vi "Single HWSync.vi"() -> ()   [LabVIEW 2014]
doc: "Use this template to build a producer/consumer design pattern with events to produce queue items. Use this design pattern instead of the User Interface Event Handler pattern for user interfaces when you want to execute code asynchronously in response to an event without slowing the user interface responsiveness."
uses:
  TypeDefs/HAL Config Data.ctl
  APIs/Data Queue/Acquisition Data 1 Sample Cluster.ctl
  APIs/Data Queue/Control Data Cluster.ctl
  APIs/Message Queue/Enqueue Message (Array).vi
  APIs/Message Queue/WINFAS 2 Message Queue.lvlib
  HWSyncLoop/HWSyncLoop.lvlib
  APIs/Data Queue/WINFAS 2 Data Queue.lvlib
panel:
  in  "Config":bool
  in  "LOAD DRIVER":bool
  in  "Disconnect":bool
  in  "Connect":bool
  in  "Sequence:Stop":bool
  in  "Sequence:Start":bool
  in  "Auto-Refresh:Stop":bool
  in  "Auto-Refresh:Start":bool
  in  "Stop Cycle":bool
  in  "Stop Measurement":bool
  in  "Start Measurement":bool
  in  "Start Cycle":bool
  out "TDX":sgl[][](graph)
  out "Valores TDX":sgl[](array[numeric]) format="%0+10.6fmm"
  out "TDX N°":i32[](array[numeric])
  in  "Encoder Zero":bool
  out "DO":bool[][](array[boolean])
  out "DI":bool[][](array[boolean])
  in  "DO Button":bool[][](array[boolean])=[[FALSE, FALSE, FALSE, FALSE, FALSE, FALSE, FALSE, FALSE], [FALSE, FALSE, FALSE, FALSE, FALSE, FALSE, FALSE, FALSE]]
  out "Encoder":sgl(knob) scale=-360.0..360.0 scale format="%.0f°"
  out "Errores":string
  out "Status Bar":string="LOAD"
  out "Driver:":string
  # "Loop para 1 Hardware Síncrono"
  # "Entradas Digitales (0-15)"
  # "Salidas Digitales (0-15)"
  # "Salidas Digitales (0-15)"
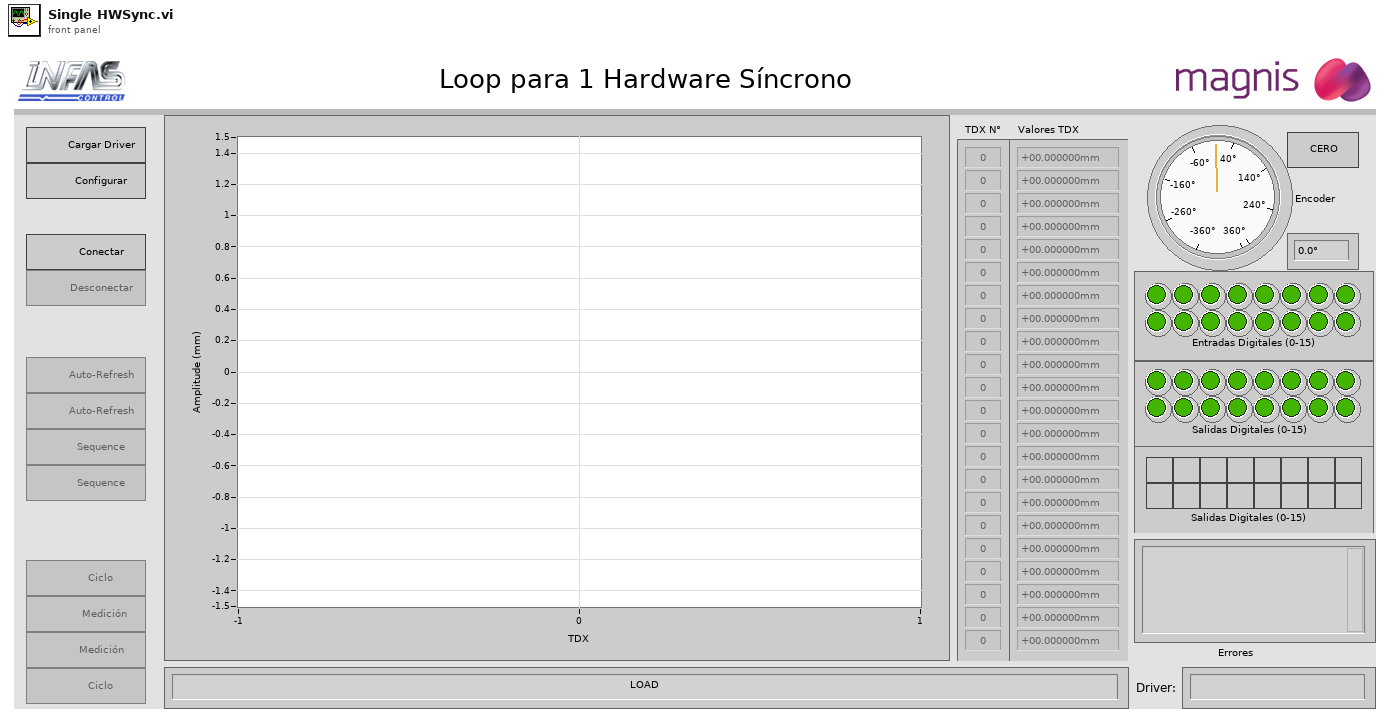
[diagram p1: front panel]
types:
  T1 = typedef "HAL Config Data.ctl" = cluster{"HWSync Index":u32, "Driver Name":string, "Channel Mask":u64}
  T2 = enum8{"Enabled", "Disabled", "Disabled and Grayed Out"}
  T3 = cluster{"LOAD DRIVER":refnum<vi>, "Config":refnum<vi>, "Connect":refnum<vi>, "Disconnect":refnum<vi>, "Auto-Refresh:Start":refnum<vi>, "Auto-Refresh:Stop":refnum<vi>, "Sequence:Start":refnum<vi>, "Sequence:Stop":refnum<vi>, "Start Cycle":refnum<vi>, "Start Measurement":refnum<vi>, "Stop Measurement":refnum<vi>, "Stop Cycle":refnum<vi>}
  T4 = enum32{"invalid app kind", "Development System", "Run Time System", "Student Edition", "Embedded LabVIEW", "Evaluation", "Custom"}
  T5 = typedef "WINFAS 2 Message Queue.lvlib/All Message Queues.ctl" = cluster{"CORE":refnum<queue>, "Event UI":refnum<queue>, "Display UI":refnum<queue>, "MATH":refnum<queue>, "SEQ":refnum<queue>, "DB":refnum<queue>, "ERR":refnum<queue>, "HAL":refnum<queue>, "HWSync1":refnum<queue>, "HWSync2":refnum<queue>, "HWSync3":refnum<queue>, "HWSync4":refnum<queue>, "HWSync5":refnum<queue>, "HWAsync1":refnum<queue>, "HWAsync2":refnum<queue>, "HWAsync3":refnum<queue>, "HWAsync4":refnum<queue>, "HWAsync5":refnum<queue>, "HWAsync6":refnum<queue>, "HWAsync7":refnum<queue>, "HWAsync8":refnum<queue>, "HWAsync9":refnum<queue>, "HWAsync10":refnum<queue>}
  T6 = typedef "WINFAS 2 Data Queue.lvlib/All Data Queues Cluster.ctl" = cluster{"Queues":cluster{"ACQ HWSync1":refnum<queue>, "ACQ HWSync2":refnum<queue>, "ACQ HWSync3":refnum<queue>, "ACQ HWSync4":refnum<queue>, "ACQ HWSync5":refnum<queue>}, "Notifiers":cluster{"Control":cluster{"CTRL HWSync1":refnum<notifier>, "CTRL HWSync2":refnum<notifier>, "CTRL HWSync3":refnum<notifier>, "CTRL HWSync4":refnum<notifier>, "CTRL HWSync5":refnum<notifier>}, "Acquisition":cluster{"ACQ HWSync1":refnum<notifier>, "ACQ HWSync2":refnum<notifier>, "ACQ HWSync3":refnum<notifier>, "ACQ HWSync4":refnum<notifier>, "ACQ HWSync5":refnum<notifier>}, "Async":cluster{"ACQ HWAsync1":refnum<notifier>, "ACQ HWAsync2":refnum<notifier>, "ACQ HWAsync3":refnum<notifier>, "ACQ HWAsync4":refnum<notifier>, "ACQ HWAsync5":refnum<notifier>, "ACQ HWAsync6":refnum<notifier>, "ACQ HWAsync7":refnum<notifier>, "ACQ HWAsync8":refnum<notifier>, "ACQ HWAsync9":refnum<notifier>, "ACQ HWAsync10":refnum<notifier>}}}
  T7 = typedef "WINFAS 2 Data Queue.lvlib/Acquisition Data 1 Sample Cluster.ctl" = cluster{"TDX":sgl[], "Encoder":sgl}
  T8 = typedef "WINFAS 2 Data Queue.lvlib/Control Data Cluster.ctl" = cluster{"Encoder":sgl, "DI":bool[], "DO":bool[]}
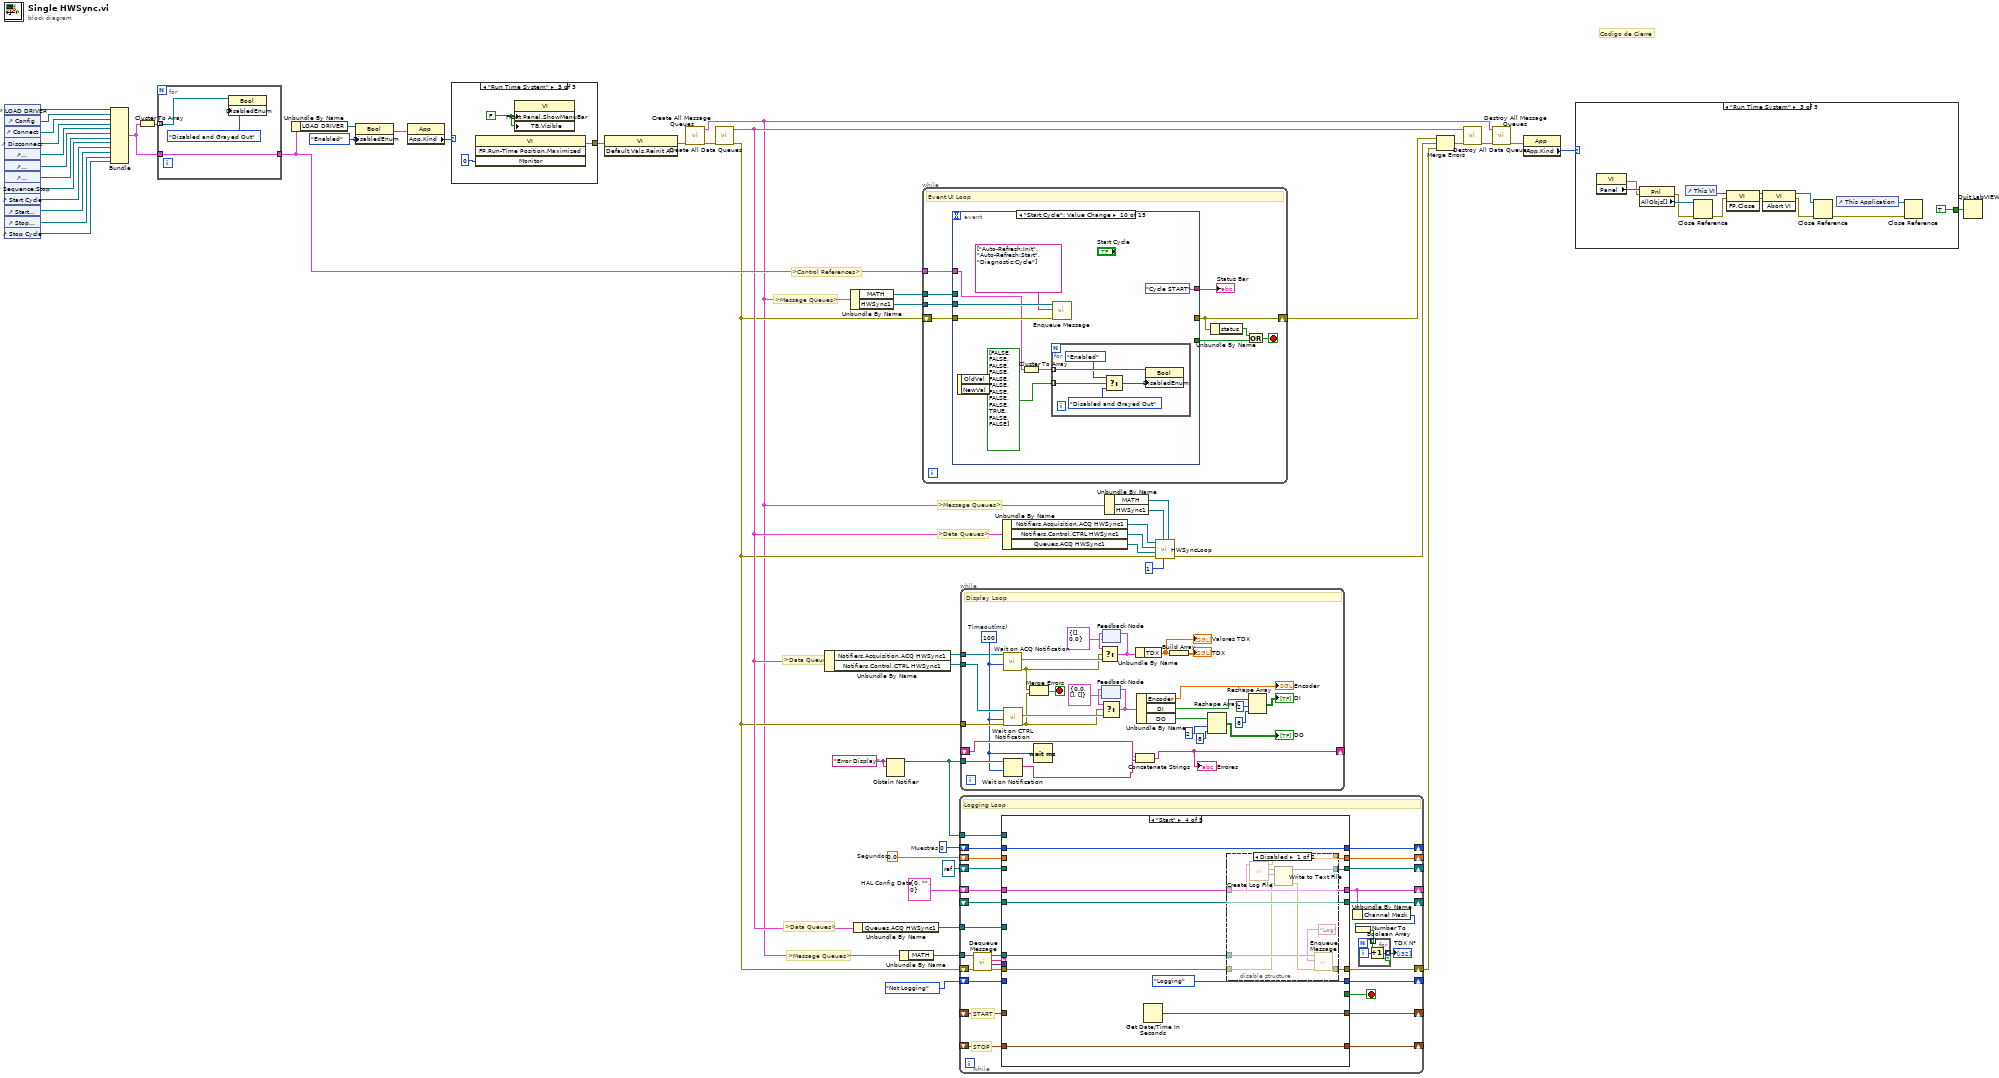
[diagram p0: block diagram]
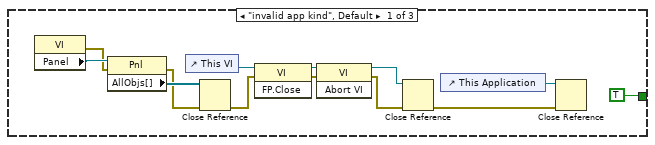
[diagram p4: hidden frame]
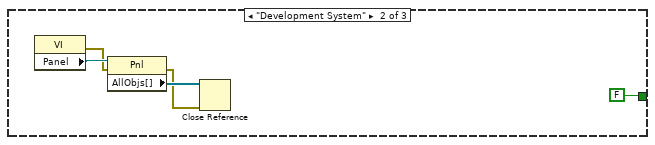
[diagram p5: hidden frame]
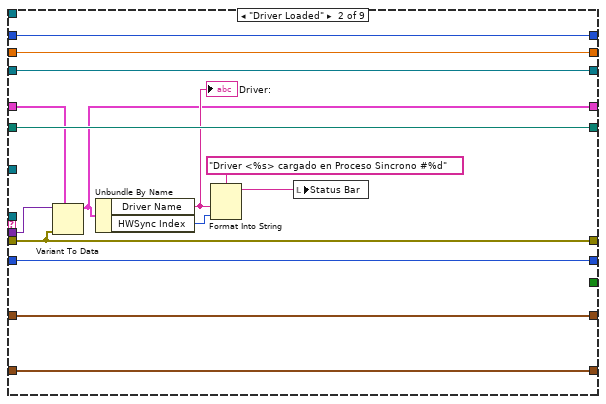
[diagram p7: hidden frame]
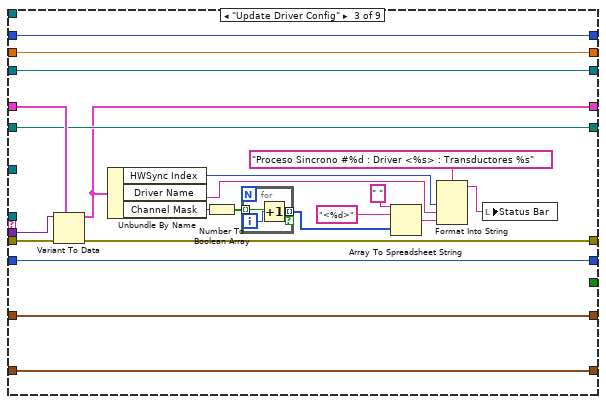
[diagram p8: hidden frame]
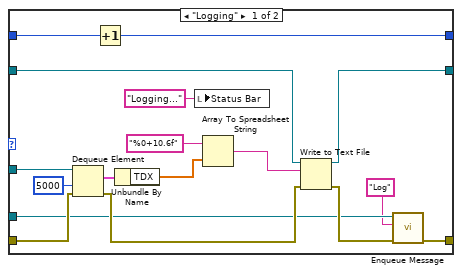
[diagram p11: hidden frame]
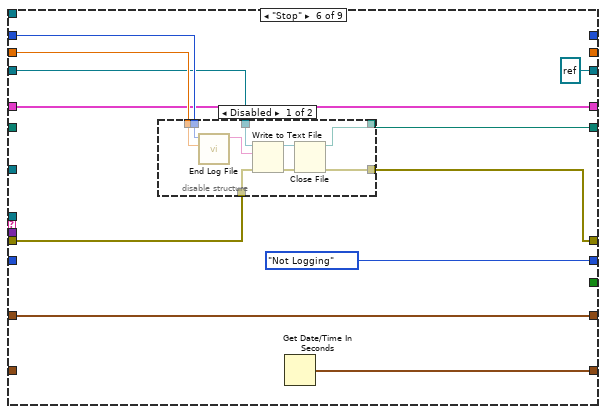
[diagram p12: hidden frame]
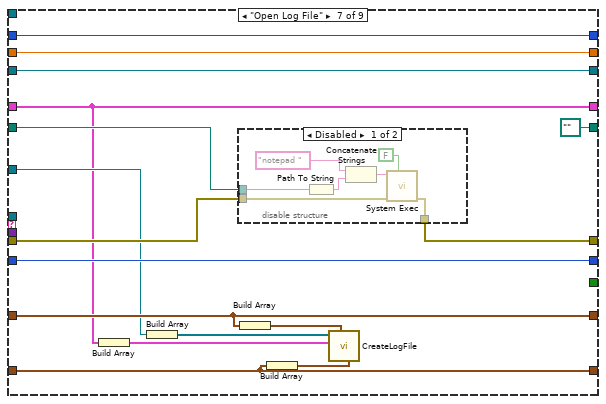
[diagram p14: hidden frame]
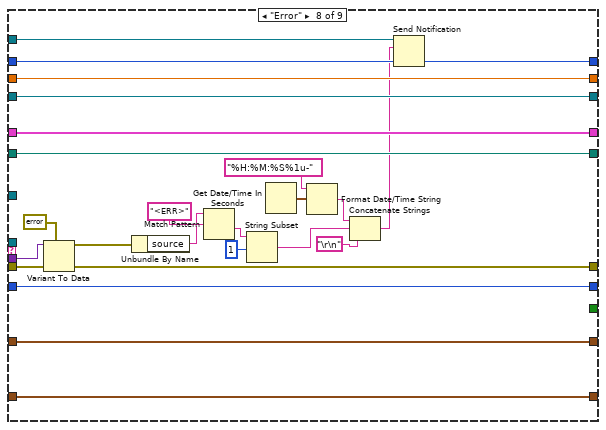
[diagram p16: hidden frame]
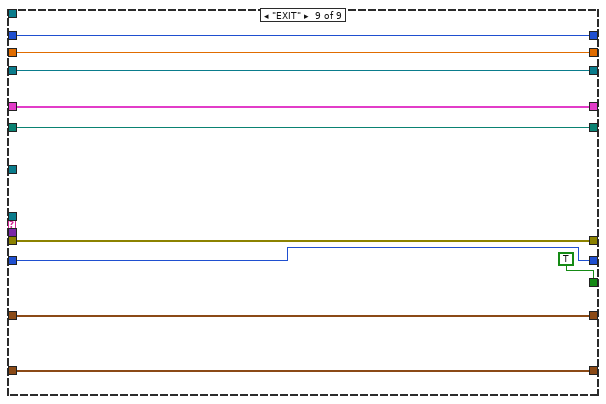
[diagram p17: hidden frame]
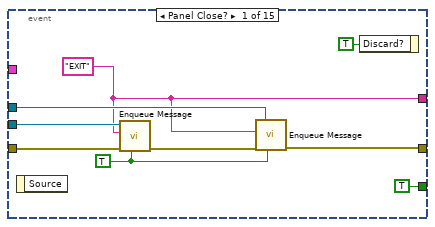
[diagram p18: hidden frame]
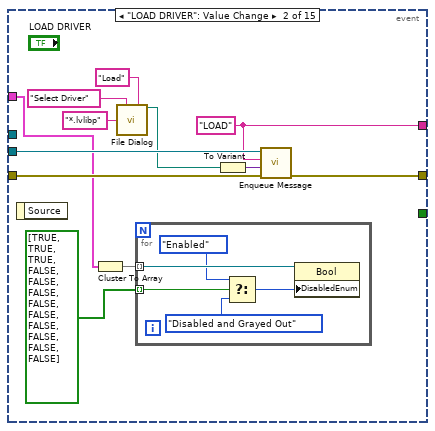
[diagram p19: hidden frame]
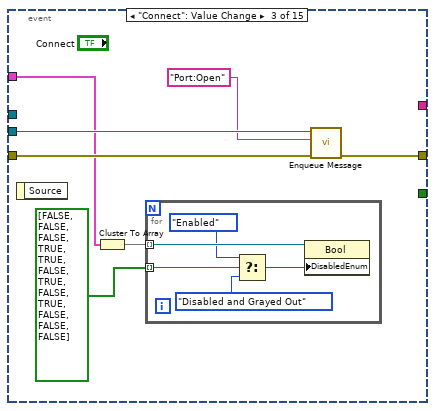
[diagram p20: hidden frame]
diagram:
  w2 = "Error Display" ("name (unnamed)")
  w11 = T1 {"HWSync Index"=0, "Driver Name"="", "Channel Mask"=0}  # HAL Config Data
  w43 = 0.0  # Segundos
  w44 = 0  # Muestras
  # ">Control References>"
  # "Codigo de Cierre"
  # ">Message Queues>"
  # ">Data Queues>"
  # ">Message Queues>"
  # ">Data Queues>"
  # ">Data Queues>"
  # ">Message Queues>"
  n1 = control-ref of="LOAD DRIVER"() -> (w14:refnum<vi>)
  n2 = control-ref of="Config"() -> (w8:refnum<vi>)
  n3 = control-ref of="Connect"() -> (w9:refnum<vi>)
  n4 = control-ref of="Disconnect"() -> (w10:refnum<vi>)
  n5 = control-ref of="Auto-Refresh:Start"() -> (w41:refnum<vi>)
  n6 = control-ref of="Auto-Refresh:Stop"() -> (w40:refnum<vi>)
  n7 = control-ref of="Sequence:Start"() -> (w39:refnum<vi>)
  n8 = control-ref of="Sequence:Stop"() -> (w38:refnum<vi>)
  n9 = control-ref of="Start Cycle"() -> (w6:refnum<vi>)
  n10 = control-ref of="Start Measurement"() -> (w5:refnum<vi>)
  n11 = control-ref of="Stop Measurement"() -> (w4:refnum<vi>)
  n12 = control-ref of="Stop Cycle"() -> (w3:refnum<vi>)
  n13 = Bundle("LOAD DRIVER"=w14, "Config"=w8, "Connect"=w9, "Disconnect"=w10, "Auto-Refresh:Start"=w41, "Auto-Refresh:Stop"=w40, "Sequence:Start"=w39, "Sequence:Stop"=w38, "Start Cycle"=w6, "Start Measurement"=w5, "Stop Measurement"=w4, "Stop Cycle"=w3) -> (w36:T3)  [unwired: 1 in]
  n14 = Cluster To Array(cluster=w36) -> (array=w37:refnum<vi>[])
  n15 = for {
    tunnel: w37 -> [w55] mode=indexing
    tunnel: w36 -> [w54]
    tunnel: [w54] -> w35
    n16 = property class="Bool"(reference=w55, "DisabledEnum"=T2."Disabled and Grayed Out" ("Disabled")) -> ()  [unwired: 1 in, 2 out]
  }
  n17 = Unbundle By Name(w35) -> ("LOAD DRIVER"=w34:refnum<vi>)
  n18 = property class="Bool"(reference=w34, "DisabledEnum"=T2."Enabled" ("Disabled")) -> (error out=w22:errorcluster)  [unwired: 1 in, 1 out]
  n19 = property class="App"(error in=w22) -> ("App.Kind"=w30:T4)  [unwired: 1 in, 2 out]
  n20 = case shown="\"Run Time System\"" w30 {
    tunnel: [_ _ w57] -> w29
    frame "invalid app kind", Default {
    }
    frame "Development System" {
    }
    frame "Run Time System" {
      w56 = FALSE ("Front Panel Window:Show Menu Bar")
      n21 = invoke class="VI" method="FP.Run-Time Position.Maximized"("Monitor"=i16 0) -> (error out=w57:errorcluster)  [unwired: 3 in, 3 out]
      n22 = property class="VI"("Front Panel.ShowMenuBar"=w56, "TB.Visible"=w56) -> ()  [unwired: 2 in, 2 out]
    }
  }
  n23 = invoke class="VI" method="Default Vals.Reinit All"(error in=w29) -> (error out=w16:errorcluster)  [unwired: 2 in, 2 out]
  n24 = call "Create All Message Queues.vi"("error in (no error)"=w16) -> ("error out"=w18:errorcluster, "Message Queues Out"=w12:T5)  [unwired: 9 in]
  n25 = call "Create All Data Queues.vi"("Error In"=w18) -> ("Error Out"=w13:errorcluster, "WINFAS 2 Data Queue.lvlib:All Data Queues Cluster"=w17:T6)  [unwired: 9 in]
  n26 = Unbundle By Name(w17) -> ("Notifiers.Acquisition.ACQ HWSync1"=w25:refnum<notifier>, "Notifiers.Control.CTRL HWSync1"=w24:refnum<notifier>)
  n27 = Unbundle By Name(w12) -> ("MATH"=w52:refnum<queue>, "HWSync1"=w48:refnum<queue>)
  n28 = Unbundle By Name(w17) -> ("Queues.ACQ HWSync1"=w23:refnum<queue>)
  n29 = Obtain Notifier(name (unnamed)=w2, notification data type=w2) -> (notifier out=w1:refnum<notifier>)  [unwired: 2 in, 2 out]
  n30 = Unbundle By Name(w12) -> ("MATH"=w45:refnum<queue>)
  n31 = while {
    shift-right: [w64] -> w49
    shift-left: w13 -> [w66]
    tunnel: w52 -> [w67]
    tunnel: w48 -> [w62]
    tunnel: w35 -> [w59]
    stop <- w60 stop-if-true
    # "Event UI Loop"
    n32 = event shown="[9] \"Start Cycle\": Value Change" {
      selector: _ -> [_ _ _ _ _ _ _ _ _ _ _ _ _ _ _]
      dyn-events: _ -> [_ _ _ _ _ _ _ _ _ _ _ _ _ _ _]
      timeout: _ -> [_ _ _ _ _ _ _ _ _ _ _ _ _ _ _]
      tunnel: w67 -> [w73 _ _ _ _ _ _ w159 w170 _ w200 w218 w235 _ _]
      tunnel: w66 -> [w75 w88 w100 w112 w120 w131 w144 w162 w178 w190 w207 w225 w242 w252 w260]
      tunnel: [w70 w86 w99 w111 w119 w127 w142 w161 w169 _ w201 w219 w236 w248 w259] -> w64
      tunnel: [TRUE ("stop") _ _ _ _ _ _ _ _ _ _ _ _ _ _] -> w65
      tunnel: w62 -> [w76 w87 w98 w110 w121 w130 w143 w160 w176 w189 w206 w224 w241 w250 w262]
      tunnel: [w72 w80 _ _ w118 w126 w141 w154 w174 "Cycle START" ("Message") "Measurement START" ("Message") "Measurement Stop" ("Message") "Cycle Stop" ("Message") _ _] -> w61
      tunnel: w59 -> [_ w79 w94 w106 _ w122 w137 w150 w171 w184 w196 w213 w231 _ _]
      event Panel Close? {
        w74 = TRUE ("Priority Message? (F)")
        w72 = "EXIT" ("String")
        n33 = event-data() -> ()  [unwired: 1 in, 1 out]
        n34 = call-poly "Enqueue Message.vi"("Priority Message? (F)"=w74, "error in (no error)"=w75, "Message"=w72, "Message Queue"=w76) -> ("error out"=w71:errorcluster)  [unwired: 6 in, 1 out]
        n35 = call-poly "Enqueue Message.vi"("Priority Message? (F)"=w74, "error in (no error)"=w71, "Message"=w72, "Message Queue"=w73) -> ("error out"=w70:errorcluster)  [unwired: 6 in, 1 out]
        n36 = event-data("Discard?"=TRUE) -> ()  [unwired: 1 in, 1 out]
      }
      event "LOAD DRIVER": Value Change {
        w80 = "LOAD" ("Message")
        n37 = event-data() -> ()  [unwired: 1 in, 1 out]
        n38 = Cluster To Array(cluster=w79) -> (array=w78:refnum<vi>[])
        n39 = call "File Dialog"("prompt"="Select Driver", "button label"="Load", "default name"="*.lvlibp") -> ("selected path"=w81:path)  [unwired: 9 in, 3 out]
        n40 = for {
          tunnel: w78 -> [w93] mode=indexing
          tunnel: bool[] [TRUE, TRUE, TRUE, FALSE, FALSE, FALSE, FALSE, FALSE, FALSE, FALSE, FALSE, FALSE] -> [w92] mode=indexing
          n41 = Select(t=T2."Enabled" ("Disabled"), s=w92, f=T2."Disabled and Grayed Out" ("Disabled")) -> (s? t:f=w89:T2)
          n42 = property class="Bool"(reference=w93, "DisabledEnum"=w89) -> ()  [unwired: 1 in, 2 out]
        }
        n43 = To Variant(anything=w81) -> (Variant=w85:variant)
        n44 = call-poly "Enqueue Message.vi"("error in (no error)"=w88, "Message Data"=w85, "Message"=w80, "Message Queue"=w87) -> ("error out"=w86:errorcluster)  [unwired: 6 in, 1 out]
      }
      event "Connect": Value Change {
        n45 = event-data() -> ()  [unwired: 1 in, 1 out]
        n46 = Cluster To Array(cluster=w94) -> (array=w96:refnum<vi>[])
        n47 = for {
          tunnel: w96 -> [w105] mode=indexing
          tunnel: bool[] [FALSE, FALSE, FALSE, TRUE, TRUE, FALSE, TRUE, FALSE, TRUE, FALSE, FALSE, FALSE] -> [w104] mode=indexing
          n48 = Select(t=T2."Enabled" ("Disabled"), s=w104, f=T2."Disabled and Grayed Out" ("Disabled")) -> (s? t:f=w101:T2)
          n49 = property class="Bool"(reference=w105, "DisabledEnum"=w101) -> ()  [unwired: 1 in, 2 out]
        }
        n50 = call-poly "Enqueue Message.vi"("error in (no error)"=w100, "Message"="Port:Open" ("String"), "Message Queue"=w98) -> ("error out"=w99:errorcluster)  [unwired: 7 in, 1 out]
      }
      event "Disconnect": Value Change {
        n51 = event-data() -> ()  [unwired: 1 in, 1 out]
        n52 = Cluster To Array(cluster=w106) -> (array=w108:refnum<vi>[])
        n53 = for {
          tunnel: w108 -> [w117] mode=indexing
          tunnel: bool[] [TRUE, TRUE, TRUE, FALSE, FALSE, FALSE, FALSE, FALSE, FALSE] -> [w116] mode=indexing
          n54 = Select(t=T2."Enabled" ("Disabled"), s=w116, f=T2."Disabled and Grayed Out" ("Disabled")) -> (s? t:f=w113:T2)
          n55 = property class="Bool"(reference=w117, "DisabledEnum"=w113) -> ()  [unwired: 1 in, 2 out]
        }
        n56 = call-poly "Enqueue Message.vi"("error in (no error)"=w112, "Message"="Port:Close" ("String"), "Message Queue"=w110) -> ("error out"=w111:errorcluster)  [unwired: 7 in, 1 out]
      }
      event "Config": Value Change {
        w118 = "Config" ("String")
        n57 = event-data() -> ()  [unwired: 1 in, 1 out]
        n58 = call-poly "Enqueue Message.vi"("error in (no error)"=w120, "Message"=w118, "Message Queue"=w121) -> ("error out"=w119:errorcluster)  [unwired: 7 in, 1 out]
      }
      event "Auto-Refresh:Start": Value Change {
        w126 = "Auto-Refresh:Start" ("Message")
        n59 = event-data() -> ()  [unwired: 1 in, 1 out]
        n60 = Cluster To Array(cluster=w122) -> (array=w124:refnum<vi>[])
        n61 = for {
          tunnel: w124 -> [w136] mode=indexing
          tunnel: bool[] [FALSE, FALSE, FALSE, FALSE, FALSE, TRUE, FALSE, FALSE, FALSE, FALSE, FALSE, FALSE] -> [w135] mode=indexing
          n62 = Select(t=T2."Enabled" ("Disabled"), s=w135, f=T2."Disabled and Grayed Out" ("Disabled")) -> (s? t:f=w132:T2)
          n63 = property class="Bool"(reference=w136, "DisabledEnum"=w132) -> ()  [unwired: 1 in, 2 out]
        }
        n64 = call-poly "Enqueue Message.vi"("error in (no error)"=w131, "Message"="Auto-Refresh:Init" ("String"), "Message Queue"=w130) -> ("error out"=w128:errorcluster, "dup Message Queue"=w125:refnum<queue>)  [unwired: 7 in]
        n65 = call-poly "Enqueue Message.vi"("error in (no error)"=w128, "Message"=w126, "Message Queue"=w125) -> ("error out"=w127:errorcluster)  [unwired: 7 in, 1 out]
      }
      event "Auto-Refresh:Stop": Value Change {
        w141 = "Auto-Refresh:Stop" ("Message")
        n66 = event-data() -> ()  [unwired: 1 in, 1 out]
        n67 = Cluster To Array(cluster=w137) -> (array=w139:refnum<vi>[])
        n68 = for {
          tunnel: w139 -> [w149] mode=indexing
          tunnel: bool[] [FALSE, FALSE, FALSE, TRUE, TRUE, FALSE, TRUE, FALSE, TRUE, FALSE, FALSE, FALSE] -> [w148] mode=indexing
          n69 = Select(t=T2."Enabled" ("Disabled"), s=w148, f=T2."Disabled and Grayed Out" ("Disabled")) -> (s? t:f=w145:T2)
          n70 = property class="Bool"(reference=w149, "DisabledEnum"=w145) -> ()  [unwired: 1 in, 2 out]
        }
        n71 = call-poly "Enqueue Message.vi"("Priority Message? (F)"=TRUE, "error in (no error)"=w144, "Message"=w141, "Message Queue"=w143) -> ("error out"=w142:errorcluster)  [unwired: 6 in, 1 out]
      }
      event "Sequence:Start": Value Change {
        w154 = "Sequence:Start" ("Message")
        n72 = event-data() -> ()  [unwired: 1 in, 1 out]
        n73 = Cluster To Array(cluster=w150) -> (array=w152:refnum<vi>[])
        n74 = for {
          tunnel: w152 -> [w167] mode=indexing
          tunnel: bool[] [FALSE, FALSE, FALSE, FALSE, FALSE, FALSE, FALSE, TRUE, FALSE, FALSE, FALSE, FALSE] -> [w166] mode=indexing
          n75 = Select(t=T2."Enabled" ("Disabled"), s=w166, f=T2."Disabled and Grayed Out" ("Disabled")) -> (s? t:f=w163:T2)
          n76 = property class="Bool"(reference=w167, "DisabledEnum"=w163) -> ()  [unwired: 1 in, 2 out]
        }
        n77 = call-poly "Enqueue Message.vi"("error in (no error)"=w162, "Message"="Sequence:Init" ("String"), "Message Queue"=w160) -> ("error out"=w157:errorcluster, "dup Message Queue"=w153:refnum<queue>)  [unwired: 7 in]
        n78 = call-poly "Enqueue Message.vi"("error in (no error)"=w157, "Message"=w154, "Message Queue"=w153) -> ("error out"=w156:errorcluster)  [unwired: 7 in, 1 out]
        n79 = call-poly "Enqueue Message.vi"("error in (no error)"=w156, "Message"="Start", "Message Queue"=w159) -> ("error out"=w161:errorcluster)  [unwired: 7 in, 1 out]
      }
      event "Sequence:Stop": Value Change {
        w174 = "Sequence:Stop" ("Message")
        n80 = event-data() -> ()  [unwired: 1 in, 1 out]
        n81 = Cluster To Array(cluster=w171) -> (array=w173:refnum<vi>[])
        n82 = for {
          tunnel: w173 -> [w183] mode=indexing
          tunnel: bool[] [FALSE, FALSE, FALSE, TRUE, TRUE, FALSE, TRUE, FALSE, TRUE, FALSE, FALSE, FALSE] -> [w182] mode=indexing
          n83 = Select(t=T2."Enabled" ("Disabled"), s=w182, f=T2."Disabled and Grayed Out" ("Disabled")) -> (s? t:f=w179:T2)
          n84 = property class="Bool"(reference=w183, "DisabledEnum"=w179) -> ()  [unwired: 1 in, 2 out]
        }
        n85 = call-poly "Enqueue Message.vi"("Priority Message? (F)"=TRUE, "error in (no error)"=w178, "Message"=w174, "Message Queue"=w176) -> ("error out"=w177:errorcluster)  [unwired: 6 in, 1 out]
        n86 = call-poly "Enqueue Message.vi"("error in (no error)"=w177, "Message Array"=string[] ["Stop", "Open Log File"], "Message Queue"=w170) -> ("error out"=w169:errorcluster)  [unwired: 7 in, 1 out]
      }
      event "Start Cycle": Value Change {
        n87 = event-data() -> ()  [unwired: 1 in, 2 out]
        n88 = Cluster To Array(cluster=w184) -> (array=w186:refnum<vi>[])
        n89 = for {
          tunnel: w186 -> [w195] mode=indexing
          tunnel: bool[] [FALSE, FALSE, FALSE, FALSE, FALSE, FALSE, FALSE, FALSE, FALSE, TRUE, FALSE, FALSE] -> [w194] mode=indexing
          n90 = Select(t=T2."Enabled" ("Disabled"), s=w194, f=T2."Disabled and Grayed Out" ("Disabled")) -> (s? t:f=w191:T2)
          n91 = property class="Bool"(reference=w195, "DisabledEnum"=w191) -> ()  [unwired: 1 in, 2 out]
        }
        n92 = call-poly "Enqueue Message.vi"("error in (no error)"=w190, "Message Array"=string[] ["Auto-Refresh:Init", "Auto-Refresh:Start", "Diagnostic:Cycle"], "Message Queue"=w189) -> ()  [unwired: 7 in, 2 out]
      }
      event "Start Measurement": Value Change {
        n93 = event-data() -> ()  [unwired: 1 in, 6 out]
        n94 = Cluster To Array(cluster=w196) -> (array=w198:refnum<vi>[])
        n95 = for {
          tunnel: w198 -> [w212] mode=indexing
          tunnel: bool[] [FALSE, FALSE, FALSE, FALSE, FALSE, FALSE, FALSE, FALSE, FALSE, FALSE, TRUE, FALSE] -> [w211] mode=indexing
          n96 = Select(t=T2."Enabled" ("Disabled"), s=w211, f=T2."Disabled and Grayed Out" ("Disabled")) -> (s? t:f=w208:T2)
          n97 = property class="Bool"(reference=w212, "DisabledEnum"=w208) -> ()  [unwired: 1 in, 2 out]
        }
        n98 = call-poly "Enqueue Message.vi"("Priority Message? Array"=bool[] [TRUE, FALSE, FALSE, FALSE], "error in (no error)"=w207, "Message Array"=string[] ["Auto-Refresh:Stop", "Sequence:Init", "Sequence:Start", "Diagnostic:Measurement"], "Message Queue"=w206) -> ("error out"=w202:errorcluster)  [unwired: 6 in, 1 out]
        n99 = call-poly "Enqueue Message.vi"("error in (no error)"=w202, "Message"="Start", "Message Queue"=w200) -> ("error out"=w201:errorcluster)  [unwired: 7 in, 1 out]
      }
      event "Stop Measurement": Value Change {
        n100 = event-data() -> ()  [unwired: 1 in, 6 out]
        n101 = Cluster To Array(cluster=w213) -> (array=w215:refnum<vi>[])
        n102 = for {
          tunnel: w215 -> [w230] mode=indexing
          tunnel: bool[] [FALSE, FALSE, FALSE, FALSE, FALSE, FALSE, FALSE, FALSE, FALSE, FALSE, FALSE, TRUE] -> [w229] mode=indexing
          n103 = Select(t=T2."Enabled" ("Disabled"), s=w229, f=T2."Disabled and Grayed Out" ("Disabled")) -> (s? t:f=w226:T2)
          n104 = property class="Bool"(reference=w230, "DisabledEnum"=w226) -> ()  [unwired: 1 in, 2 out]
        }
        n105 = call-poly "Enqueue Message.vi"("Priority Message? Array"=bool[] [TRUE, FALSE, FALSE], "error in (no error)"=w225, "Message Array"=string[] ["Sequence:Stop", "Auto-Refresh:Init", "Auto-Refresh:Start"], "Message Queue"=w224) -> ("error out"=w220:errorcluster)  [unwired: 6 in, 1 out]
        n106 = call-poly "Enqueue Message.vi"("Priority Message? (F)"=TRUE, "error in (no error)"=w220, "Message"="Stop", "Message Queue"=w218) -> ("error out"=w219:errorcluster)  [unwired: 6 in, 1 out]
      }
      event "Stop Cycle": Value Change {
        n107 = event-data() -> ()  [unwired: 1 in, 6 out]
        n108 = Cluster To Array(cluster=w231) -> (array=w233:refnum<vi>[])
        n109 = for {
          tunnel: w233 -> [w247] mode=indexing
          tunnel: bool[] [FALSE, FALSE, FALSE, TRUE, TRUE, FALSE, TRUE, FALSE, TRUE, FALSE, FALSE, FALSE] -> [w246] mode=indexing
          n110 = Select(t=T2."Enabled" ("Disabled"), s=w246, f=T2."Disabled and Grayed Out" ("Disabled")) -> (s? t:f=w243:T2)
          n111 = property class="Bool"(reference=w247, "DisabledEnum"=w243) -> ()  [unwired: 1 in, 2 out]
        }
        n112 = call-poly "Enqueue Message.vi"("Priority Message? Array"=bool[] [TRUE], "error in (no error)"=w242, "Message Array"=string[] ["Auto-Refresh:Stop"], "Message Queue"=w241) -> ("error out"=w237:errorcluster)  [unwired: 6 in, 1 out]
        n113 = call-poly "Enqueue Message.vi"("error in (no error)"=w237, "Message"="Open Log File", "Message Queue"=w235) -> ("error out"=w236:errorcluster)  [unwired: 7 in, 1 out]
      }
      event "Encoder Zero": Value Change {
        n114 = event-data() -> ()  [unwired: 1 in, 6 out]
        n115 = call-poly "Enqueue Message.vi"("Priority Message? (F)"=TRUE, "error in (no error)"=w252, "Message"="Encoder Zero", "Message Queue"=w250) -> ("error out"=w248:errorcluster)  [unwired: 6 in, 1 out]
      }
      event "DO Button": Value Change {
        n116 = event-data() -> ()  [unwired: 1 in, 1 out]
        n117 = Reshape Array("DO Button", 16 ("dimension size")) -> (w253:bool[])
        n118 = Boolean Array To Number(Boolean array=w253) -> (number=w256:u32)
        n119 = To Variant(anything=w256) -> (Variant=w257:variant)
        n120 = call "Enqueue Message (Single).vi"("Priority Message? (F)"=TRUE, "error in (no error)"=w260, "Message Data"=w257, "Message"="Digital Out Write", "Message Queue"=w262) -> ("error out"=w259:errorcluster)  [unwired: 5 in, 1 out]
      }
    }
    "Status Bar" <- w61
    n121 = Unbundle By Name(w64) -> ("status"=w63:bool)
    n122 = Or(x=w63, y=w65) -> (x .or. y?=w60:bool)
  }
  n123 = while {
    tunnel: w23 -> [w288]
    tunnel: w45 -> [w287]
    shift-right: [w290] -> _
    shift-left: refnum<file> refnum ("refnum out") -> [w289]
    shift-right: [w284] -> w15
    shift-left: w13 -> [w283]
    shift-right: [w282] -> _
    shift-left: w43 -> [w281]
    shift-right: [w280] -> _
    shift-left: w44 -> [w279]
    shift-right: [w270] -> _
    shift-left: w11 -> [w277]
    shift-right: [w275] -> _
    shift-left: _ -> [w274]
    shift-right: [w272] -> _
    shift-left: enum16{"Logging", "Not Logging"}."Not Logging" -> [w273]
    tunnel: w1 -> [w271]
    shift-right: [w266] -> _
    shift-left: _ -> [w265]
    shift-right: [w264] -> _
    shift-left: _ -> [w263]
    stop <- w286 stop-if-true
    # "STOP"
    # "START"
    # "Logging Loop"
    n124 = call "Dequeue Message.vi"("error in (no error)"=w283, "Message Queue"=w287) -> ("error out"=w285:errorcluster, "Message Data"=w276:variant, "Message"=w291:string, "dup Message Queue"=w278:refnum<queue>)  [unwired: 6 in]
    n125 = case shown="\"Start\"" w291 {
      tunnel: [w303 w318 w340 w354 w376 refnum<file> refnum ("refnum out") w434 w460 w475] -> w290
      tunnel: w289 -> [w303 w318 w340 _ w377 w406 w434 w460 w475]
      tunnel: w288 -> [_ _ _ _ w378 _ w422 _ _]
      tunnel: w278 -> [_ _ _ w353 w373 _ _ _ _]
      tunnel: [_ _ _ _ _ _ _ _ TRUE] -> w286
      tunnel: w285 -> [w302 w313 w337 w349 w375 w402 w431 w458 w473]
      tunnel: [w302 w313 w336 w352 w374 w403 w430 w456 w473] -> w284
      tunnel: [w300 w317 w339 w351 w372 _ w433 w465 w471] -> w282
      tunnel: w281 -> [w300 w317 w339 _ w372 w408 w433 w465 w471]
      tunnel: [w301 w316 w338 w350 w370 _ w432 w464 w472] -> w280
      tunnel: w279 -> [w301 w316 w338 w350 w371 w407 w432 w464 w472]
      tunnel: w277 -> [w299 w307 w335 w348 w369 w405 w420 w462 w470]
      tunnel: [w299 w306 w331 w348 w369 w405 w420 w462 w470] -> w270
      tunnel: w276 -> [_ w312 w334 _ _ _ _ w459 _]
      tunnel: [w298 w315 w333 w347 w368 w404 path "" ("path") w463 w469] -> w275
      tunnel: w274 -> [w298 w315 w333 w347 w368 _ w429 w463 w469]
      tunnel: w273 -> [w297 w314 w332 _ w367 _ w427 w461 w468]
      tunnel: [w297 w314 w332 enum16{"Logging", "Not Logging"}."Logging" w367 enum16{"Logging", "Not Logging"}."Not Logging" w427 w461 w468] -> w272
      tunnel: w271 -> [_ _ _ _ _ _ _ w445 _]
      tunnel: [w296 w305 w320 w345 w366 w400 w426 w443 w467] -> w266
      tunnel: w265 -> [w296 w305 w320 _ w366 w400 w426 w443 w467]
      tunnel: [w295 w304 w319 w344 w365 w399 w425 w442 w466] -> w264
      tunnel: w263 -> [w295 w304 w319 w344 w365 _ w425 w442 w466]
      frame Default {
      }
      frame "Driver Loaded" {
        n126 = Variant To Data(error in=w313, type=w307, Variant=w312) -> (data=w306:T1)  [unwired: 1 out]
        n127 = Unbundle By Name(w306) -> ("Driver Name"=w308:string, "HWSync Index"=w309:u32)
        "Driver:" <- w308
        n128 = Format Into String(format string="Driver <%s> cargado en Proceso Sincrono #%d", w308, w309) -> (resulting string=w310:string)  [unwired: 2 in, 1 out]
        n129 = local write "Status Bar"(w310) -> ()
      }
      frame "Update Driver Config" {
        n130 = Variant To Data(error in=w337, type=w335, Variant=w334) -> (data=w331:T1, error out=w336:errorcluster)
        n131 = Unbundle By Name(w331) -> ("HWSync Index"=w329:u32, "Driver Name"=w328:string, "Channel Mask"=w326:u64)
        n132 = Number To Boolean Array(number=w326) -> (Boolean array=w325:bool[])
        n133 = for {
          tunnel: w325 -> [w341] mode=indexing
          tunnel: [w342] -> w324 mode=indexing if=w341
          i -> [w343]
          n134 = Increment(x=w343) -> (x+1=w342:i32)
        }
        n135 = Array To Spreadsheet String(delimiter (Tab)=" ", array=w324, 3:"<%d>" ("format string")) -> (spreadsheet string=w322:string)
        n136 = Format Into String(format string="Proceso Sincrono #%d : Driver <%s> : Transductores %s", w329, w328, w322) -> (resulting string=w327:string)  [unwired: 2 in, 1 out]
        n137 = local write "Status Bar"(w327) -> ()
      }
      frame "Start" {
        n138 = Get Date/Time In Seconds() -> (seconds since 1Jan1904=w345:timestamp)
        n139 = disable-structure shown="Disabled" {
          disable-tunnel: [w364 _] -> w354
          disable-tunnel: w353 -> [w362 _]
          disable-tunnel: [w360 _] -> w352
          disable-tunnel: [w359 _] -> w351
          disable-tunnel: w349 -> [w356 _]
          disable-tunnel: w348 -> [w355 _]
          frame Disabled {
            n140 = call "Create Log File.vi"("HAL Config Data"=w355) -> ("String"=w357:string, "Byte Stream File out"=w358:refnum<file>, "Seconds"=w359:dbl)  [unwired: 8 in]
            n141 = Write to Text File(file (use dialog)=w358, text=w357, error in=w356) -> (refnum out=w364:refnum<file>, error out=w363:errorcluster)  [unwired: 1 in, 1 out]
            n142 = call-poly "Enqueue Message.vi"("error in (no error)"=w363, "Message"="Log", "Message Queue"=w362) -> ("error out"=w360:errorcluster)  [unwired: 7 in, 1 out]
          }
          frame Enabled {
          }
        }
      }
      frame "Log" {
        n143 = case shown="\"Not Logging\", Default" w367 {
          tunnel: w378 -> [w395 _]
          tunnel: w377 -> [w393 w397]
          tunnel: [w392 w397] -> w376
          tunnel: w375 -> [w391 w396]
          tunnel: [w387 w396] -> w374
          tunnel: w373 -> [w386 _]
          tunnel: w371 -> [w384 w398]
          tunnel: [w382 w398] -> w370
          frame "Logging" {
            n144 = Dequeue Element(queue=w395, timeout in ms (-1)=5000, error in (no error)=w391) -> (element=w394:T7, error out=w390:errorcluster)  [unwired: 2 out]
            n145 = Increment(x=w384) -> (x+1=w382:i32)
            n146 = Unbundle By Name(w394) -> ("TDX"=w381:sgl[])
            n147 = local write "Status Bar"("Logging..." ("Status Bar")) -> ()
            n148 = Array To Spreadsheet String(array=w381, 3:"%0+10.6f" ("format string")) -> (spreadsheet string=w379:string)  [unwired: 1 in]
            n149 = Write to Text File(file (use dialog)=w393, text=w379, error in=w390) -> (refnum out=w392:refnum<file>, error out=w388:errorcluster)  [unwired: 1 in, 1 out]
            n150 = call-poly "Enqueue Message.vi"("error in (no error)"=w388, "Message"="Log", "Message Queue"=w386) -> ("error out"=w387:errorcluster)  [unwired: 7 in, 1 out]
          }
          frame "Not Logging", Default {
          }
        }
      }
      frame "Stop" {
        n151 = disable-structure shown="Disabled" {
          disable-tunnel: w408 -> [w417 _]
          disable-tunnel: w407 -> [w416 _]
          disable-tunnel: w406 -> [w414 _]
          disable-tunnel: [w412 _] -> w404
          disable-tunnel: [w411 _] -> w403
          disable-tunnel: w402 -> [w410 _]
          frame Disabled {
            n152 = call "End Log File.vi"("Seconds"=w417, "Muestras totales"=w416) -> ("String"=w415:string)  [unwired: 9 in]
            n153 = Write to Text File(file (use dialog)=w414, text=w415, error in=w410) -> (refnum out=w418:refnum<file>, error out=w413:errorcluster)  [unwired: 1 in, 1 out]
            n154 = Close File(refnum=w418, error in=w413) -> (path=w412:path, error out=w411:errorcluster)
          }
          frame Enabled {
          }
        }
        n155 = Get Date/Time In Seconds() -> (seconds since 1Jan1904=w399:timestamp)
      }
      frame "Open Log File" {
        n156 = Build Array(w420) -> (w419:T1[])
        n157 = Build Array(w422) -> (w421:refnum<queue>[])
        n158 = disable-structure shown="Disabled" {
          disable-tunnel: w431 -> [w437 _]
          disable-tunnel: [w436 _] -> w430
          disable-tunnel: w429 -> [w435 _]
          frame Disabled {
            n159 = Path To String(path=w435) -> (string=w440:string)
            n160 = Concatenate Strings("notepad ", w440) -> (w438:string)
            n161 = call <vilib>:"System Exec.vi"("wait until completion? (T)"=FALSE, "error in (no error)"=w437, "command line"=w438) -> ("error out"=w436:errorcluster)  [unwired: 5 in, 3 out]
          }
          frame Enabled {
          }
        }
        n162 = Build Array(w426) -> (w424:timestamp[])
        n163 = Build Array(w425) -> (w423:timestamp[])
        n164 = call "CreateLogFile.vi"("Stop Time"=w423, "Start Time"=w424, "HAL Config"=w419, "ACQ Queues"=w421) -> ()  [unwired: 8 in]
      }
      frame "Error" {
        n165 = Variant To Data(error in=w458, type=errorcluster {"status"=FALSE, "code"=0, "source"=""} ("error out"), Variant=w459) -> (data=w455:errorcluster, error out=w456:errorcluster)
        n166 = Unbundle By Name(w455) -> ("source"=w453:string)
        n167 = Match Pattern(string=w453, regular expression="<ERR>") -> (after substring=w448:string)  [unwired: 1 in, 3 out]
        n168 = String Subset(string=w448, offset (0)=1) -> (substring=w447:string)  [unwired: 1 in]
        n169 = Get Date/Time In Seconds() -> (seconds since 1Jan1904=w452:timestamp)
        n170 = Format Date/Time String(time format string (%c)="%H:%M:%S%1u-", seconds (now)=w452) -> (date/time string=w449:string)  [unwired: 1 in]
        n171 = Concatenate Strings(w449, w447, "\r\n") -> (w444:string)
        n172 = Send Notification(notification=w444, notifier=w445) -> ()  [unwired: 1 in, 2 out]
      }
      frame "EXIT" {
      }
    }
    n173 = Unbundle By Name(w270) -> ("Channel Mask"=w269:u64)
    n174 = Number To Boolean Array(number=w269) -> (Boolean array=w268:bool[])
    n175 = for {
      tunnel: w268 -> [w292] mode=indexing
      tunnel: [w293] -> w267 mode=indexing if=w292
      i -> [w294]
      n176 = Increment(x=w294) -> (x+1=w293:i32)
    }
    "TDX N°" <- w267
  }
  n177 = while {
    tunnel: w25 -> [w476]
    tunnel: w24 -> [w500]
    tunnel: w13 -> [w492]
    tunnel: w1 -> [w482]
    shift-right: [w480] -> _
    shift-left: _ -> [w481]
    stop <- w493 stop-if-true
    w477 = 100  # Timeout(ms)
    # "Display Loop"
    n178 = call "Wait on ACQ Notification.vi"("timeout in ms (-1)"=w477, "ACQ Data Notifier in"=w476) -> ("error out"=w488:errorcluster, "1 Sample"=w496:T7)  [unwired: 6 in, 2 out]
    n179 = call "Wait on CTRL Notification.vi"("error in (no error)"=w492, "timeout in ms (-1)"=w477, "CTRL Data Notifier in"=w500) -> ("error out"=w489:errorcluster, "Control Data"=w499:T8)  [unwired: 5 in, 2 out]
    n180 = Wait on Notification(notifier=w482, timeout in ms (-1)=w477) -> (notification=w478:string)  [unwired: 2 in, 3 out]
    n181 = Merge Errors(w488, w489) -> (w493:errorcluster)
    n182 = Wait (ms)(milliseconds to wait=w477) -> ()  [unwired: 1 out]
    n183 = feedback #1(T8 {"Encoder"=0.0, "DI"=[], "DO"=[]} ("Control Data")) -> (w498:T8)
    n184 = Select(t=w498, s=w489, f=w499) -> (s? t:f=w497:T8)
    n185 = feedback-in #1(w497) -> ()
    n186 = feedback #2(T7 {"TDX"=[], "Encoder"=0.0} ("1 Sample")) -> (w495:T7)
    n187 = Select(t=w495, s=w488, f=w496) -> (s? t:f=w494:T7)
    n188 = feedback-in #2(w494) -> ()
    n189 = Unbundle By Name(w494) -> ("TDX"=w479:sgl[])
    "Valores TDX" <- w479
    n190 = Concatenate Strings(w478, w481) -> (w480:string)
    "Errores" <- w480
    n191 = Unbundle By Name(w497) -> ("Encoder"=→"Encoder":sgl, "DI"=w505:bool[], "DO"=w502:bool[])
    n192 = Build Array(w479) -> (→"TDX":sgl[][])
    n193 = Reshape Array(w502, 2 ("index"), 8 ("dimension size")) -> (→"DO":bool[][])
    n194 = Reshape Array(w505, 2 ("index"), 8 ("dimension size")) -> (→"DI":bool[][])
  }
  n195 = Unbundle By Name(w17) -> ("Notifiers.Acquisition.ACQ HWSync1"=w28:refnum<notifier>, "Notifiers.Control.CTRL HWSync1"=w27:refnum<notifier>, "Queues.ACQ HWSync1"=w26:refnum<queue>)
  n196 = Unbundle By Name(w12) -> ("MATH"=w51:refnum<queue>, "HWSync1"=w50:refnum<queue>)
  n197 = call "HWSyncLoop.vi"("HAL"=w51, "Index"=u32 1 ("Num of Loop"), "HWSync"=w50, "error in"=w13, "ACQ Data Queue"=w26, "CTRL Data Notifier"=w27, "ACQ Data Notifier"=w28) -> ("error out"=w47:errorcluster)  [unwired: 4 in]
  n198 = Merge Errors(w49, w47, w15) -> (w21:errorcluster)
  n199 = call "Destroy All Data Queues.vi"("Error In"=w21, "WINFAS 2 Data Queue.lvlib:All Data Queues Cluster"=w17) -> ("Error Out"=w20:errorcluster)  [unwired: 9 in]
  n200 = call "Destroy All Message Queues.vi"("error in (no error)"=w20, "Message Queues Out"=w12) -> ("error out"=w19:errorcluster)  [unwired: 9 in]
  n201 = property class="App"(error in=w19) -> ("App.Kind"=w32:T4)  [unwired: 1 in, 2 out]
  n202 = case shown="\"Run Time System\"" w32 {
    tunnel: [TRUE FALSE TRUE] -> w31
    frame "invalid app kind", Default {
      n203 = property class="VI"() -> (error out=w506:errorcluster, "Panel"=w516:refnum<vi>)  [unwired: 2 in, 1 out]
      n204 = property class="Pnl"(reference=w516, error in=w506) -> (error out=w507:errorcluster, "AllObjs[]"=w515:refnum<vi>[])  [unwired: 1 out]
      n205 = control-ref of="This VI"() -> (w513:refnum<vi>)
      n206 = Close Reference(reference=w515, error in (no error)=w507) -> (error out=w512:errorcluster)
      n207 = invoke class="VI" method="FP.Close"(reference=w513, error in=w512) -> (reference out=w511:refnum<vi>, error out=w510:errorcluster)  [unwired: 1 in, 1 out]
      n208 = invoke class="VI" method="Abort VI"(reference=w511, error in=w510) -> (reference out=w508:refnum<vi>, error out=w509:errorcluster)  [unwired: 1 in, 1 out]
      n209 = Close Reference(reference=w508, error in (no error)=w509) -> (error out=w517:errorcluster)
      n210 = control-ref of="This Application"() -> (w518:refnum<vi>)
      n211 = Close Reference(reference=w518, error in (no error)=w517) -> ()  [unwired: 1 out]
    }
    frame "Development System" {
      n212 = property class="VI"() -> (error out=w519:errorcluster, "Panel"=w523:refnum<vi>)  [unwired: 2 in, 1 out]
      n213 = property class="Pnl"(reference=w523, error in=w519) -> (error out=w520:errorcluster, "AllObjs[]"=w522:refnum<vi>[])  [unwired: 1 out]
      n214 = Close Reference(reference=w522, error in (no error)=w520) -> ()  [unwired: 1 out]
    }
    frame "Run Time System" {
      n215 = property class="VI"() -> (error out=w524:errorcluster, "Panel"=w534:refnum<vi>)  [unwired: 2 in, 1 out]
      n216 = property class="Pnl"(reference=w534, error in=w524) -> (error out=w525:errorcluster, "AllObjs[]"=w533:refnum<vi>[])  [unwired: 1 out]
      n217 = control-ref of="This VI"() -> (w531:refnum<vi>)
      n218 = Close Reference(reference=w533, error in (no error)=w525) -> (error out=w530:errorcluster)
      n219 = invoke class="VI" method="FP.Close"(reference=w531, error in=w530) -> (reference out=w529:refnum<vi>, error out=w528:errorcluster)  [unwired: 1 in, 1 out]
      n220 = invoke class="VI" method="Abort VI"(reference=w529, error in=w528) -> (reference out=w526:refnum<vi>, error out=w527:errorcluster)  [unwired: 1 in, 1 out]
      n221 = Close Reference(reference=w526, error in (no error)=w527) -> (error out=w535:errorcluster)
      n222 = control-ref of="This Application"() -> (w536:refnum<vi>)
      n223 = Close Reference(reference=w536, error in (no error)=w535) -> ()  [unwired: 1 out]
    }
  }
  n224 = Quit LabVIEW(quit? (T)=w31) -> ()
